vi "supported actions list template.vi"() -> (3 "supported actions list":T1[](array[typedef]))   [LabVIEW 2014, in "Simple Sequencer TBM editor node.lvclass"]
doc: "This VI provides an interface for exposing the list of actions that the sequencer can interact with. VIs must return an array of clusters containing the configuration class for the action, the display name of the action, and the UI VI path for that action."
uses:
  Simple Sequencer TBM editor node.lvclass
  action config and UI pairing.ctl
  sequencer parent classes/action configuration parent/action configuration.lvclass
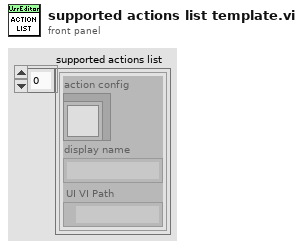
[diagram p1: front panel]
types:
  T1 = typedef "Simple Sequencer TBM editor node.lvclass/action config and UI pairing.ctl" = cluster{"action config":refnum<class "action configuration.lvclass">, "display name":string, "UI VI Path":path}
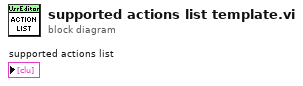
[diagram p0: block diagram]
diagram:
